vi "Steering Encoder (RAW to Final).vi"(1 "offsets[]":dbl[](array[numeric]), 2 "encoderRAW[]":dbl[](array[numeric])) -> (0 "finalAngle":dbl[](array[numeric]))   [LabVIEW 2019]
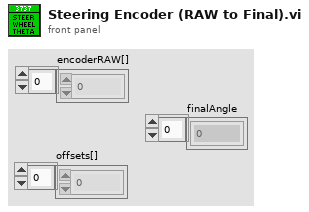
[diagram p1: front panel]
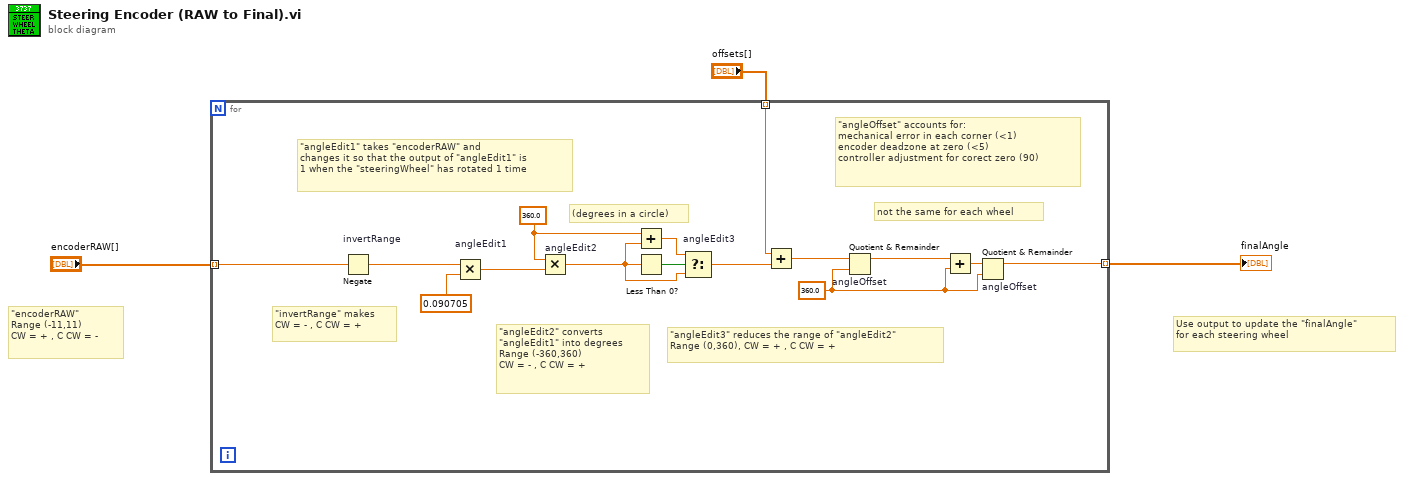
[diagram p0: block diagram]
diagram:
  # "Use output to update the \"finalAngle\"\nfor each steering wheel"
  # "\"encoderRAW\"\nRange (-11,11)\nCW = + , C CW = -"
  n1 = for {
    tunnel: "encoderRAW[]" -> [w9] mode=indexing
    tunnel: [w8] -> w2 mode=indexing
    tunnel: "offsets[]" -> [w7] mode=indexing
    w5 = 360.0
    w11 = 360.0 ("x")
    # "not the same for each wheel"
    # "\"angleOffset\" accounts for:\nmechanical error in each corner (<1)\nencoder deadzone at zero (<5)\ncontroller adjustment for corect zero (90)"
    # "(degrees in a circle)"
    # "\"angleEdit3\" reduces the range of \"angleEdit2\"\nRange (0,360), CW = + , C CW = +"
    # "\"invertRange\" makes\nCW = - , C CW = +"
    # "\"angleEdit2\" converts\n\"angleEdit1\" into degrees\nRange (-360,360)\nCW = - , C CW = +"
    # "\"angleEdit1\" takes \"encoderRAW\" and\nchanges it so that the output of \"angleEdit1\" is\n1 when the \"steeringWheel\" has rotated 1 time"
    n2 = Negate "invertRange"(x=w9) -> (-x=w14:dbl)
    n3 = Multiply "angleEdit1"(x=w14, y=0.090705) -> (x*y=w12:dbl)
    n4 = Multiply "angleEdit2"(x=w11, y=w12) -> (x*y=w15:dbl)
    n5 = Add(x=w11, y=w15) -> (x+y=w16:dbl)
    n6 = Less Than 0?(x=w15) -> (x < 0?=w17:bool)
    n7 = Select "angleEdit3"(t=w16, s=w17, f=w15) -> (s? t:f=w13:dbl)
    n8 = Add ("+")(x=w7, y=w13) -> (x+y=w6:dbl)
    n9 = Quotient & Remainder "angleOffset"(x=w6, y=w5) -> (x-y*floor(x/y)=w4:dbl)  [unwired: 1 out]
    n10 = Add(x=w4, y=w5) -> (x+y=w10:dbl)
    n11 = Quotient & Remainder "angleOffset"(x=w10, y=w5) -> (x-y*floor(x/y)=w8:dbl)  [unwired: 1 out]
  }
  "finalAngle" <- w2
